vi "trajectory_FF.vi"(5 "BoundaryZpelv":dbl[](array[numeric]), 6 "BoundaryYpelv":dbl[](array[numeric]), 7 "BoundaryXPelv":dbl[](array[numeric]), 8 "pel_cn_atStanding":dbl[](array[numeric]), 9 "viconData_2":dbl[](array[numeric]), 10 "K constant_pel":dbl, 11 "FM --- FF_pel":dbl[](array[numeric])) -> (1 "DesiredFM":dbl[](array[numeric]), 2 "InsideBounds":bool)   [LabVIEW 2017]
uses:
  <vilib>/Analysis/_algsub.llb/Real Vector Norm.vi
  <vilib>/Analysis/NI_AALPro.lvlib
panel:
  out "currentpt":dbl[](array[numeric])
  out "zmax":dbl
  out "zmin":dbl
  # "INPUTS"
  # "Calculated Values:"
  # "OUTPUTS:"
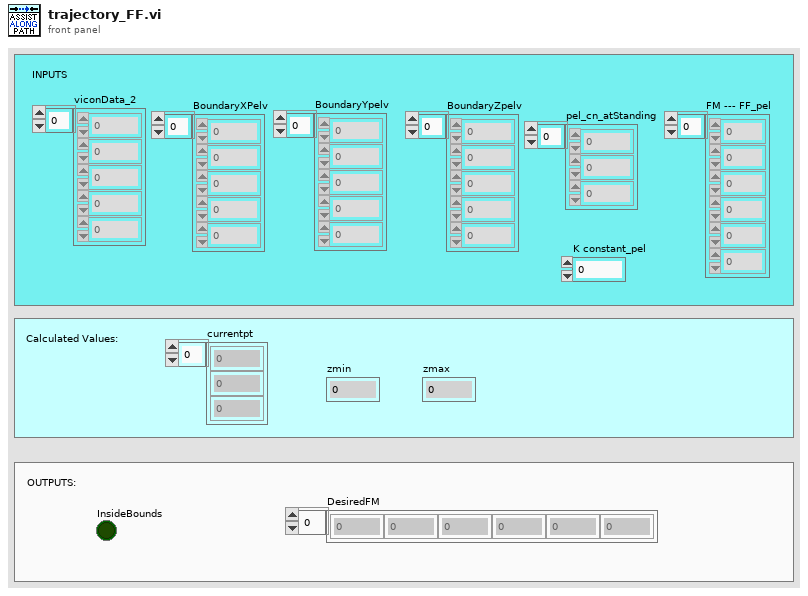
[diagram p1: front panel]
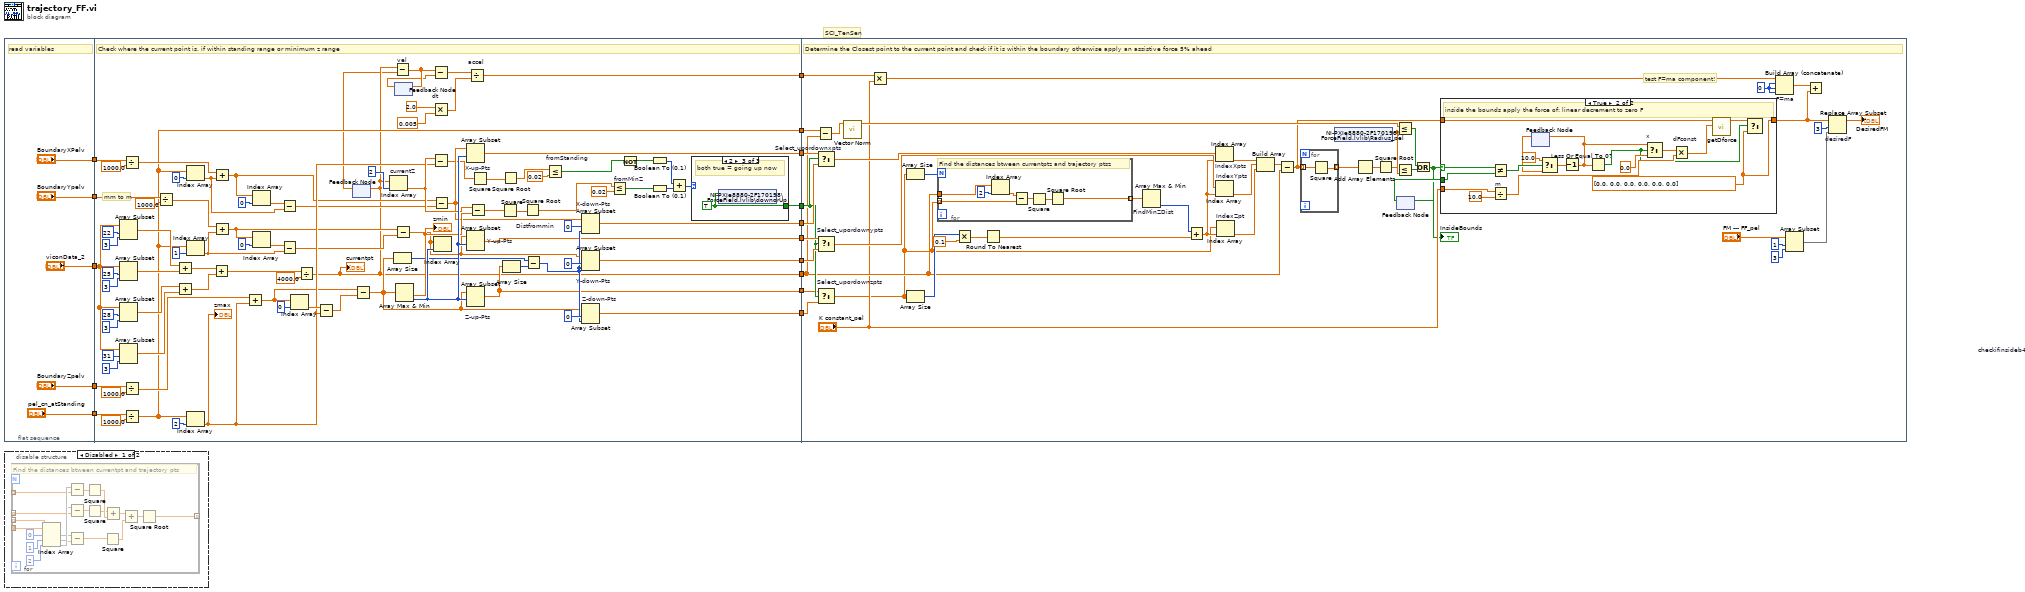
[diagram p0: block diagram]
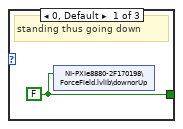
[diagram p3: hidden frame]
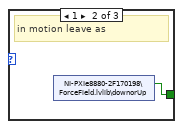
[diagram p4: hidden frame]
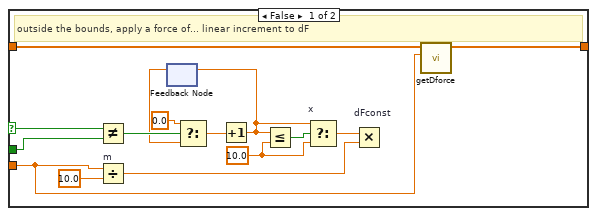
[diagram p5: hidden frame]
diagram:
  # "SCI_TenSen"
  n1 = flat-sequence {
    tunnel: ["viconData_2"] -> w15
    tunnel: ["BoundaryZpelv"] -> w14
    tunnel: ["pel_cn_atStanding"] -> w13
    tunnel: ["BoundaryYpelv"] -> w12
    tunnel: ["BoundaryXPelv"] -> w11
    tunnel: w15 -> [w94]
    tunnel: w14 -> [w88]
    tunnel: w13 -> [w51]
    tunnel: w12 -> [w85]
    tunnel: w11 -> [w82]
    tunnel: [w29] -> w10
    tunnel: [w71] -> w9
    tunnel: [w57] -> w8
    tunnel: [w70] -> w7
    tunnel: [w69] -> w6
    tunnel: [w68] -> w5
    tunnel: [w67] -> w4
    tunnel: [w66] -> w3
    tunnel: [w50] -> w2
    tunnel: [w21] -> w1
    tunnel: w10 -> [w133]
    tunnel: w9 -> [w159]
    tunnel: w8 -> [w154]
    tunnel: w7 -> [w158]
    tunnel: w6 -> [w157]
    tunnel: w5 -> [w156]
    tunnel: w4 -> [w155]
    tunnel: w3 -> [w153]
    tunnel: w2 -> [w134]
    tunnel: w1 -> [w125]
    frame #0 {
      # "read variables"
    }
    frame #1 {
      # "mm to m"
      # "Check where the current point is, if within standing range or minimum z range"
      n2 = Array Subset(array=w94, index=22, length=3) -> (w104:dbl[])
      n3 = Array Subset(array=w94, index=25, length=3) -> (w105:dbl[])
      n4 = Array Subset(array=w94, index=28, length=3) -> (w106:dbl[])
      n5 = Array Subset(array=w94, index=31, length=3) -> (w107:dbl[])
      n6 = Divide(x=w82, y=1000.0) -> (x/y=w81:dbl[])
      n7 = Divide(x=w88, y=1000.0) -> (x/y=w89:dbl[])
      n8 = Divide(x=w51, y=1000.0) -> (x/y=w50:dbl[])
      n9 = Divide(x=w85, y=1000.0) -> (x/y=w86:dbl[])
      n10 = Add(x=w104, y=w105) -> (x+y=w109:dbl[])
      n11 = Add(x=w106, y=w107) -> (x+y=w108:dbl[])
      n12 = Index Array(array=w50, index=0) -> (element=w37:dbl)
      n13 = Index Array(array=w50, index=1) -> (element=w34:dbl)
      n14 = Index Array(array=w50, index=2) -> (element=w46:dbl)
      "zmax" <- w46
      n15 = Add(x=w109, y=w108) -> (x+y=w110:dbl[])
      n16 = Add(x=w81, y=w37) -> (x+y=w38:dbl[])
      n17 = Add(x=w86, y=w34) -> (x+y=w32:dbl[])
      n18 = Add(x=w89, y=w46) -> (x+y=w45:dbl[])
      n19 = Index Array(array=w38, index=0) -> (element=w41:dbl)
      n20 = Index Array(array=w32, index=0) -> (element=w36:dbl)
      n21 = Subtract(x=w41, y=w37) -> (x-y=w40:dbl)
      n22 = Subtract(x=w36, y=w34) -> (x-y=w33:dbl)
      n23 = Index Array(array=w45, index=0) -> (element=w47:dbl)
      n24 = Divide(x=w110, y=4000.0) -> (x/y=w29:dbl[])
      "currentpt" <- w29
      n25 = Subtract(x=w47, y=w46) -> (x-y=w44:dbl)
      n26 = feedback-in #1(w29) -> ()
      n27 = feedback #1() -> (w28:dbl[])  [unwired: 1 in]
      n28 = Subtract(x=w45, y=w44) -> (x-y=w43:dbl[])
      n29 = Index Array "currentZ"(array=w29, index=2) -> (element=w53:dbl)
      n30 = Array Size(array=w43) -> (size(s)=w49:i32)
      n31 = Subtract "vel"(x=w29, y=w28) -> (x-y=w27:dbl[])
      n32 = feedback #2() -> (w26:dbl[])  [unwired: 1 in]
      n33 = feedback-in #2(w27) -> ()
      n34 = Subtract(x=w32, y=w33) -> (x-y=w31:dbl[])
      n35 = Array Max & Min(array=w43) -> (min value=w55:dbl, min index (indices)=w72:i32)  [unwired: 2 out]
      "zmin" <- w55
      n36 = Subtract ("accel")(x=w27, y=w26) -> (x-y=w25:dbl[])
      n37 = Multiply "dt"(x=2.0, y=0.005) -> (x*y=w24:dbl)
      n38 = Subtract(x=w53, y=w46) -> (x-y=w30:dbl)
      n39 = Subtract(x=w38, y=w40) -> (x-y=w39:dbl[])
      n40 = Index Array(array=w31, index=w72) -> ()  [unwired: 1 out]
      n41 = Array Subset "X-up-Pts"(array=w39, index=w72) -> (w70:dbl[])  [unwired: 1 in]
      n42 = Array Subset "Y-up-Pts"(array=w31, index=w72) -> (w68:dbl[])  [unwired: 1 in]
      n43 = Array Subset "Z-up-Pts"(array=w43, index=w72) -> (w66:dbl[])  [unwired: 1 in]
      n44 = Divide "accel"(x=w25, y=w24) -> (x/y=w21:dbl[])
      n45 = Subtract(x=w53, y=w55) -> (x-y=w75:dbl)
      n46 = Square(x=w30) -> (x^2=w52:dbl)
      n47 = Square(x=w75) -> (x^2=w54:dbl)
      n48 = Square Root(x=w52) -> (sqrt(x)=w65:dbl)
      n49 = Array Size(array=w66) -> (size(s)=w79:i32)
      n50 = Square Root "Distfrommin"(x=w54) -> (sqrt(x)=w73:dbl)
      n51 = Subtract(x=w49, y=w79) -> (x-y=w76:i32)
      n52 = Less Or Equal? "fromStanding"(x=w65, y=0.02) -> (x <= y?=w63:bool)
      n53 = Array Subset "X-down-Pts"(array=w39, index=0, length=w76) -> (w71:dbl[])
      n54 = Array Subset "Y-down-Pts"(array=w31, index=0, length=w76) -> (w69:dbl[])
      n55 = Array Subset "Z-down-Pts"(array=w43, index=0, length=w76) -> (w67:dbl[])
      n56 = Less Or Equal? "fromMinZ"(x=w73, y=0.02) -> (x <= y?=w61:bool)
      n57 = Not(x=w63) -> (.not. x?=w62:bool)
      n58 = Boolean To (0,1)(Boolean=w62) -> (0, 1=w60:i16)
      n59 = Boolean To (0,1)(Boolean=w61) -> (0, 1=w59:i16)
      n60 = Add(x=w60, y=w59) -> (x+y=w58:i16)
      n61 = case shown="2" w58 {
        tunnel: [w111 w112 w113] -> w57
        frame 0, Default {
          w111 = FALSE
          # "standing thus going down"
          n62 = shared-variable "NI-PXIe8880-2F170198\\ForceField.lvlib\\downorUp"(w111) -> ()  [unwired: 1 in, 1 out]
        }
        frame 1 {
          # "in motion leave as"
          n63 = shared-variable "NI-PXIe8880-2F170198\\ForceField.lvlib\\downorUp"() -> (w112:bool)  [unwired: 1 in, 1 out]
        }
        frame 2 {
          w113 = TRUE
          # "both true = going up now"
          n64 = shared-variable "NI-PXIe8880-2F170198\\ForceField.lvlib\\downorUp"(w113) -> ()  [unwired: 1 in, 1 out]
        }
      }
    }
    frame #2 {
      w127 = 0
      # "test F=ma component!"
      # "Determine the Closest point to the current point and check if it is within the boundary otherwise apply an assistive force 5% ahead"
      n65 = Subtract(x=w134, y=w133) -> (x-y=w132:dbl[])
      n66 = Select "Select_upordownxpts"(t=w158, s=w154, f=w159) -> (s? t:f=w151:dbl[])
      n67 = Select "Select_upordownypts"(t=w156, s=w154, f=w157) -> (s? t:f=w150:dbl[])
      n68 = Select "Select_upordownzpts"(t=w153, s=w154, f=w155) -> (s? t:f=w121:dbl[])
      n69 = call-poly <vilib>:"Vector Norm.vi"("Input Vector"=w132) -> ("norm"=w131:dbl)  [unwired: 9 in, 1 out]
      n70 = Multiply(x=w125, y="K constant_pel") -> (x*y=w123:dbl[])
      n71 = Array Size(array=w121) -> (size(s)=w152:i32)
      n72 = Array Size(array=w121) -> (size(s)=w149:i32)
      n73 = for {
        N: w152 -> [_]
        tunnel: [w201] -> w160 mode=indexing
        tunnel: w133 -> [w200]
        tunnel: w121 -> [w197] mode=indexing
        # "Find the distances btween currentptz and trajectory ptsz"
        n74 = Index Array(array=w200, index=2) -> (element=w198:dbl)
        n75 = Subtract(x=w198, y=w197) -> (x-y=w196:dbl)
        n76 = Square(x=w196) -> (x^2=w195:dbl)
        n77 = Square Root(x=w195) -> (sqrt(x)=w201:dbl)
      }
      n78 = Multiply(x=w149, y=0.1) -> (x*y=w147:dbl)
      n79 = Round To Nearest(number=w147) -> (nearest integer value=w145:dbl)
      n80 = Array Max & Min "FindMinZDist"(array=w160) -> (min index (indices)=w146:i32)  [unwired: 3 out]
      n81 = Add(x=w146, y=w145) -> (x+y=w144:dbl)
      n82 = Index Array "IndexXpts"(array=w151, index=w144) -> (element=w141:dbl)
      n83 = Index Array "IndexYpts"(array=w150, index=w144) -> (element=w142:dbl)
      n84 = Index Array "IndexZpt"(array=w121, index=w144) -> (element=w143:dbl)
      n85 = Build Array(w141, w142, w143) -> (w135:dbl[])
      n86 = Subtract(x=w135, y=w133) -> (x-y=w120:dbl[])
      n87 = for {
        tunnel: w120 -> [w162] mode=indexing
        tunnel: [w161] -> w119 mode=indexing
        n88 = Square(x=w162) -> (x^2=w161:dbl)
      }
      n89 = shared-variable "NI-PXIe8880-2F170198\\ForceField.lvlib\\Radius_pel"() -> (w130:dbl)  [unwired: 1 in, 1 out]
      n90 = Add Array Elements(numeric array=w119) -> (sum=w118:dbl)
      n91 = Square Root(x=w118) -> (sqrt(x)=w117:dbl)
      n92 = Less Or Equal?(x=w131, y=w130) -> (x <= y?=w129:bool)
      n93 = Less Or Equal?(x=w117, y=w130) -> (x <= y?=w128:bool)
      n94 = feedback #3 "checkifinsideb4"() -> (w115:bool)  [unwired: 1 in]
      n95 = Or(x=w129, y=w128) -> (x .or. y?=w114:bool)
      "InsideBounds" <- w114
      n96 = feedback-in #3(w114) -> ()
      n97 = case shown="True" w114 {
        selector: w114 -> [w175 w187]
        tunnel: w120 -> [w177 w184]
        tunnel: [w176 w179] -> w122
        tunnel: "K constant_pel" -> [w163 w186]
        tunnel: w115 -> [w164 w178]
        frame False {
          w167 = 10.0 ("y")
          # "outside the bounds, apply a force of... linear increment to dF"
          n98 = Not Equal?(x=w175, y=w164) -> (x != y?=w174:bool)
          n99 = Divide "m"(x=w163, y=10.0) -> (x/y=w165:dbl)
          n100 = feedback #4() -> (w171:dbl)  [unwired: 1 in]
          n101 = Select(t=0.0, s=w174, f=w171) -> (s? t:f=w172:dbl)
          n102 = Increment(x=w172) -> (x+1=w168:dbl)
          n103 = feedback-in #4(w168) -> ()
          n104 = Less Or Equal?(x=w168, y=w167) -> (x <= y?=w169:bool)
          n105 = Select "x"(t=w168, s=w169, f=w167) -> (s? t:f=w166:dbl)
          n106 = Multiply "dFconst"(x=w166, y=w165) -> ()  [unwired: 1 out]
          n107 = call "getDforce.vi"("ForceDesired"=w163, "Desired Direction"=w177) -> ("FX FY Fz 0 0 0"=w176:dbl[])  [unwired: 5 in]
        }
        frame True {
          w179 = dbl[] [0.0, 0.0, 0.0, 0.0, 0.0, 0.0]
          # "inside the bounds apply the force of: linear decrement to zero F"
          n108 = Not Equal?(x=w187, y=w178) -> (x != y?=w194:bool)
          n109 = Divide "m"(x=w186, y=10.0) -> (x/y=w188:dbl)
          n110 = feedback #5() -> (w191:dbl)  [unwired: 1 in]
          n111 = Select(t=10.0, s=w194, f=w191) -> (s? t:f=w192:dbl)
          n112 = Decrement(x=w192) -> (x-1=w180:dbl)
          n113 = feedback-in #5(w180) -> ()
          n114 = Less Or Equal To 0?(x=w180) -> (x <= 0?=w182:bool)
          n115 = Select "x"(t=w180, s=w182, f=0.0) -> (s? t:f=w189:dbl)
          n116 = Multiply "dFconst"(x=w189, y=w188) -> (x*y=w183:dbl)
          n117 = call "getDforce.vi"("ForceDesired"=w183, "Desired Direction"=w184) -> ("FX FY Fz 0 0 0"=w181:dbl[])  [unwired: 5 in]
          n118 = Select(t=w181, s=w182, f=w179) -> ()  [unwired: 1 out]
        }
      }
      n119 = Build Array (concatenate) "F=ma"(w123, w127, w127, w127) -> (w126:dbl[])
      n120 = Array Subset(array="FM --- FF_pel", index=1, length=3) -> (w136:dbl[])
      n121 = Add(x=w126, y=w122) -> ()  [unwired: 1 out]
      n122 = Replace Array Subset "desiredF"(array=w122, new element=w136, index=3 ("length")) -> (→"DesiredFM":dbl[])
    }
  }
  n123 = disable-structure shown="Disabled" {
    frame Disabled {
      n124 = for {
        tunnel: _ -> [w211] mode=indexing
        tunnel: [w217] -> _ mode=indexing
        tunnel: _ -> [w216]
        tunnel: _ -> [w209] mode=indexing
        tunnel: _ -> [w204] mode=indexing
        # "Find the distances btween currentpt and trajectory pts"
        n125 = Index Array(array=w216, index #1=0 ("index"), index #2=1 ("index"), index #3=2 ("index")) -> (element #1=w205, element #2=w210, element #3=w212)
        n126 = Subtract(x=w212, y=w211) -> (x-y=w220:dbl)
        n127 = Subtract(x=w210, y=w209) -> (x-y=w208:dbl)
        n128 = Subtract(x=w205, y=w204) -> (x-y=w203:dbl)
        n129 = Square(x=w220) -> (x^2=w207:dbl)
        n130 = Square(x=w208) -> (x^2=w206:dbl)
        n131 = Square(x=w203) -> (x^2=w202:dbl)
        n132 = Add(x=w206, y=w207) -> (x+y=w219:dbl)
        n133 = Add(x=w219, y=w202) -> (x+y=w218:dbl)
        n134 = Square Root(x=w218) -> (sqrt(x)=w217:dbl)
      }
    }
    frame Enabled {
    }
  }
